vi "qKLT.vi"(0 "System no.":i32=1 min=1 max=4 step=1, 2 "Start Coordinate System":string, 3 "End Coordinate System":string, 5 "error in":errorcluster) -> (14 "Response":string, 19 "error out":errorcluster)   [LabVIEW 2026]
doc: "Returns the resulting coordinate system of a chain. A chain consists of minimum two linked coordinate systems. The resulting coordinate system is calculated beginning with the first specified coordinate system. The calculation ends with the second coordinate system if specified. If no second coordinate system is specified, \"ZERO\" is used for calculation. The position of the resulting coordinate system is canonical (SPI swivel (x, y, z) = (0, 0, 0)). If no parameters are used, the positions of all coordinate systems are returned with second coordinate system \"ZERO\". End Coordinate System is only valid in combination with Start Coordinate System.\n\nC-887, F-206, M-8X0: Only for GCS syntax version = GCS 2.0 or higher (Check with CSV?.vi. If CSV?.vi is not supported, syntax version is GCS 1.0)."
panel:
  # "Returns the resulting coordinate system of a chain."
  # "Only valid in combination\nwith Start Coordinate System:"
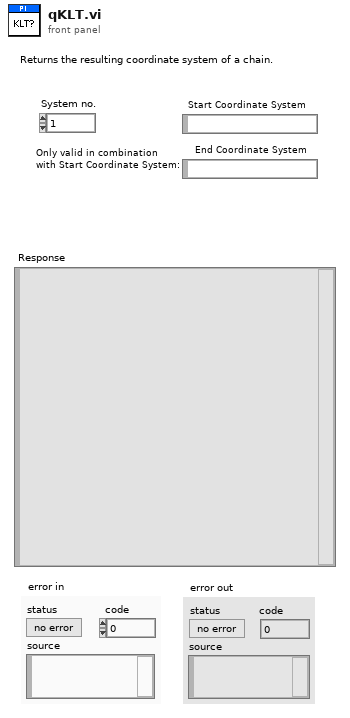
[diagram p1: front panel]
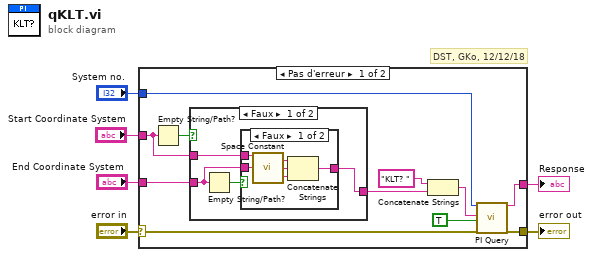
[diagram p0: block diagram]
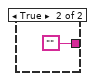
[diagram p3: hidden frame]
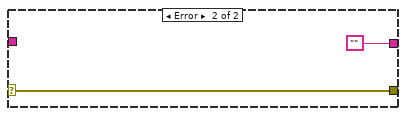
[diagram p4: hidden frame]
diagram:
  # "DST, GKo, 12/12/18"
  n1 = case shown="Pas d'erreur" "error in" {
    selector: "error in" -> [w9 w28]
    tunnel: [w8 "" ("String read")] -> w6
    tunnel: [w7 w28] -> w5
    tunnel: "System no." -> [w17 _]
    tunnel: "Start Coordinate System" -> [w11 _]
    tunnel: "End Coordinate System" -> [w14 _]
    frame No Error {
      n2 = Empty String/Path?(string/path=w11) -> (empty?=w10:bool)
      n3 = case shown="Faux" w10 {
        tunnel: w14 -> [w18 _]
        tunnel: [w21 ""] -> w13
        tunnel: w11 -> [w20 _]
        frame False {
          n4 = Empty String/Path?(string/path=w18) -> (empty?=w19:bool)
          n5 = case shown="Faux" w19 {
            tunnel: [w22 w26] -> w21
            tunnel: w20 -> [w25 w26]
            tunnel: w18 -> [w23 _]
            frame False {
              n6 = call <vilib>:"Space Constant.vi"() -> ("String"=w24:string)
              n7 = Concatenate Strings(w25, w24, w23) -> (w22:string)
            }
            frame True {
            }
          }
        }
        frame True {
        }
      }
      n8 = Concatenate Strings("KLT? " ("string"), w13) -> (w15:string)
      n9 = call "PI Query.vi"("System no."=w17, "String to send"=w15, "Attach termination char.?"=TRUE ("Attach Linefeed?"), "error in"=w9) -> ("String read"=w8:string, "error out"=w7:errorcluster)  [unwired: 3 in, 11 out]
    }
    frame Error {
    }
  }
  "Response" <- w6
  "error out" <- w5
